vi "PPR_DRIVE_Set_Wheel_Speeds.vi"(9 "Right Wheel Speed M/S":dbl format="%17.2f", 11 "Left Wheel Speed M/S":dbl format="%17.2f") -> ()   [LabVIEW 2019]
uses:
  PPR_DRIVE_GLOBALS.vi
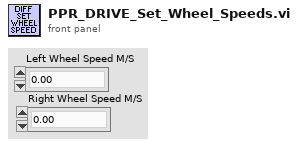
[diagram p1: front panel]
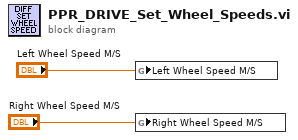
[diagram p0: block diagram]
diagram:
  n1 = global write "PPR_DRIVE_GLOBALS.vi" "Left Wheel Speed M/S"("Left Wheel Speed M/S") -> ()
  n2 = global write "PPR_DRIVE_GLOBALS.vi" "Right Wheel Speed M/S"("Right Wheel Speed M/S") -> ()
